vi "Meas Proc QWTB Set Params Table.vi"(8 "error in":errorcluster, 10 "qwtb parameters":T1[](array[typedef]), 11 "param table ref":refnum<vi>) -> (0 "error out":errorcluster)   [LabVIEW 2018]
doc: "Takes previously parsed QWTB parameters and assigns them to the parameters table. Note the parameters order must match the algorithm parameters order."
uses:
  Meas Proc QWTB Algorithm Parameter Data.ctl
panel:
  out "data":string[][](array[string])
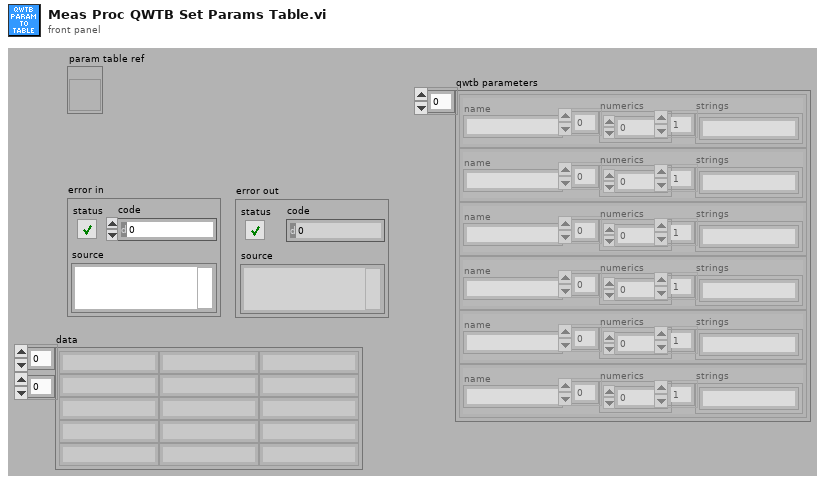
[diagram p1: front panel]
types:
  T1 = typedef "Meas Proc QWTB Algorithm Parameter Data.ctl" = cluster{"name":string, "numerics":dbl[], "strings":string[]}
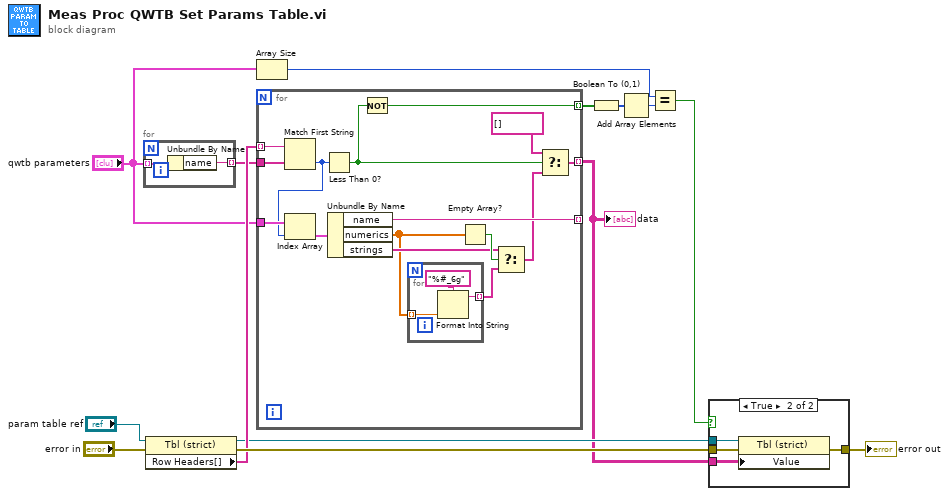
[diagram p0: block diagram]
diagram:
  n1 = for {
    tunnel: "qwtb parameters" -> [w16] mode=indexing
    tunnel: [w15] -> w8 mode=indexing
    n2 = Unbundle By Name(w16) -> ("name"=w15:string)
  }
  n3 = property class="Tbl (strict)"(reference="param table ref", error in="error in") -> (reference out=w9:refnum<vi>, error out=w12:errorcluster, "Row Headers[]"=w11:string[])
  n4 = Array Size(array="qwtb parameters") -> (size(s)=w2:i32)
  n5 = for {
    tunnel: "qwtb parameters" -> [w20]
    tunnel: [w27] -> _ mode=indexing
    tunnel: w11 -> [w26] mode=indexing
    tunnel: w8 -> [w25]
    tunnel: [w23] -> w6 mode=indexing
    tunnel: [w17] -> w7 mode=indexing
    n6 = Match First String(2:w25, 3:w26) -> (0:w19:i32)  [unwired: 1 out]
    n7 = Index Array(array=w20, index=w19) -> (element=w18:T1)
    n8 = Less Than 0?(x=w19) -> (x < 0?=w21:bool)
    n9 = Unbundle By Name(w18) -> ("name"=w27:string, "numerics"=w29:dbl[], "strings"=w30:string[])
    n10 = Not(x=w21) -> (.not. x?=w17:bool)
    n11 = for {
      tunnel: w29 -> [w34] mode=indexing
      tunnel: [w32] -> w28 mode=indexing
      n12 = Format Into String(format string="%#_6g", w34) -> (resulting string=w32:string)  [unwired: 2 in, 1 out]
    }
    n13 = Empty Array?(array=w29) -> (empty?=w31:bool)
    n14 = Select(t=w30, s=w31, f=w28) -> (s? t:f=w24:string[])
    n15 = Select(t=string[] [], s=w21, f=w24) -> (s? t:f=w23:string[])
  }
  "data" <- w6
  n16 = Boolean To (0,1)(Boolean=w7) -> (0, 1=w5:i16[])
  n17 = Add Array Elements(numeric array=w5) -> (sum=w3:i16)
  n18 = Equal?(x=w2, y=w3) -> (x = y?=w1:bool)
  n19 = case shown="True" w1 {
    tunnel: w12 -> [w35 w39]
    tunnel: w9 -> [_ w38]
    tunnel: [w35 w37] -> w14
    tunnel: w6 -> [_ w36]
    frame False {
    }
    frame True {
      n20 = property class="Tbl (strict)"(reference=w38, error in=w39, "Value"=w36) -> (error out=w37:errorcluster)  [unwired: 1 out]
    }
  }
  "error out" <- w14
